vi "StartAlbumAcq.vi"(8 "error in (no error)":errorcluster, 11 "Config In":T1={"Hardware Configuration"={"Camera Configuration"={"Setting"={"Expouse"=0.0, "Frames"=0.0, "Interval"=0.0, "ROI"={"x"=0.0, "y"=0.0, "width"=0.0, "height"=0.0}, "Binning"={"Binning X"=0.0, "Binning Y"=0.0}}, "Resource"={"CameraRef"=refnum, "LibraryRef"=refnum, "ImagesArray"=[]}}, "Stages Configuration"={"Resource"={"NanoStage Ref"=0, "MicroStage Ref"=0, "TirfLock Ref"=0}, "SettingValues"={"NanoState"={"Time"=0.0, "X"=0.0, "Y"=0.0, "Z"=0.0}, "MicroState"={"Time 2"=0.0, "Z"=0.0, "IsEPISet?"=FALSE}, "TirfLock"={"Time"=0.0, "X"=0.0, "Y"=0.0, "Sum"=0.0, "Calbrate"=0.0, "LockedTarget"=0.0, "Kp"=0.0, "Ki"=0.0, "Avg"=0.0}}}, "Lasers Configuration"={"SettingValues"={"405 Power"=0.0, "488 Power"=0.0, "532 Power"=0.0, "561 Power"=0.0, "647 Power"=0.0, "785 Power"=0.0}, "Resource"={"Library Ref"=refnum, "Lasers Ref"={"405 Ref"=refnum, "488 Ref"=refnum, "532 Ref"=refnum, "561 Ref"=refnum, "647 Ref"=refnum, "785 Ref"=refnum}}}}, "Logging Configuration"={"Log File Base Folder"=path "", "FileSurfix"="", "TiffFileFullPath"=path "", "TimeStampFile Ref"=refnum, "NoteFileRef"=refnum, "QuickNoteInfo"=""}, "HardWare Status"={"CameraAndStages"={"Camera"=FALSE, "NanoStage"=FALSE, "MicroStage"=FALSE, "TIRFLock"=FALSE}, "Lasers"={"IsConnected"={"405"=FALSE, "488"=FALSE, "532"=FALSE, "561"=FALSE, "647"=FALSE, "785"=FALSE}, "IsOpened"={"405"=FALSE, "488"=FALSE, "532"=FALSE, "561"=FALSE, "647"=FALSE, "785"=FALSE}}}, "CallBack Ref"={"LiveAcq callback Ref"=refnum, "AlbumAcq callback Ref"=refnum, "SequenceAcq callback Ref"=refnum, "Camera Status callback Ref"=refnum}, "Acqusition Control"={"Images Saving"={"StreamToDisk?"=FALSE, "SingleStack?"=FALSE, "Alert when finish?"=FALSE}, "Debug"={"Global Debug"=FALSE, "Global Debug Value"=0.0}}, "Runtime Parameters"={"Scale Bar"=TRUE, "ScaleBarSize"=10.0, "XYIncreatement+"=40.0, "ZIncreatement++"=5.0, "Autostretch"=FALSE, "ZIncreatement+"=0.2, "MicroStage+"=100.0, "XYIncreatement++"=80.0}} {"Runtime Parameters"."XYIncreatement++" format="%#_13g"; "Runtime Parameters"."MicroStage+" format="%#_13g"; "Runtime Parameters"."ZIncreatement+" format="%#_13g"; "Runtime Parameters"."ZIncreatement++" format="%#_13g"; "Runtime Parameters"."XYIncreatement+" format="%#_13g"; "Runtime Parameters"."ScaleBarSize" format="%#_13g"; "Hardware Configuration"."Lasers Configuration"."SettingValues"."785 Power" format="%.1f"; "Hardware Configuration"."Lasers Configuration"."SettingValues"."647 Power" format="%.1f"; "Hardware Configuration"."Lasers Configuration"."SettingValues"."561 Power" format="%.1f"}) -> (0 "error out":errorcluster, 3 "Config Out":T1={"Hardware Configuration"={"Camera Configuration"={"Setting"={"Expouse"=0.0, "Frames"=0.0, "Interval"=0.0, "ROI"={"x"=0.0, "y"=0.0, "width"=0.0, "height"=0.0}, "Binning"={"Binning X"=0.0, "Binning Y"=0.0}}, "Resource"={"CameraRef"=refnum, "LibraryRef"=refnum, "ImagesArray"=[]}}, "Stages Configuration"={"Resource"={"NanoStage Ref"=0, "MicroStage Ref"=0, "TirfLock Ref"=0}, "SettingValues"={"NanoState"={"Time"=0.0, "X"=0.0, "Y"=0.0, "Z"=0.0}, "MicroState"={"Time 2"=0.0, "Z"=0.0, "IsEPISet?"=FALSE}, "TirfLock"={"Time"=0.0, "X"=0.0, "Y"=0.0, "Sum"=0.0, "Calbrate"=0.0, "LockedTarget"=0.0, "Kp"=0.0, "Ki"=0.0, "Avg"=0.0}}}, "Lasers Configuration"={"SettingValues"={"405 Power"=0.0, "488 Power"=0.0, "532 Power"=0.0, "561 Power"=0.0, "647 Power"=0.0, "785 Power"=0.0}, "Resource"={"Library Ref"=refnum, "Lasers Ref"={"405 Ref"=refnum, "488 Ref"=refnum, "532 Ref"=refnum, "561 Ref"=refnum, "647 Ref"=refnum, "785 Ref"=refnum}}}}, "Logging Configuration"={"Log File Base Folder"=path "", "FileSurfix"="", "TiffFileFullPath"=path "", "TimeStampFile Ref"=refnum, "NoteFileRef"=refnum, "QuickNoteInfo"=""}, "HardWare Status"={"CameraAndStages"={"Camera"=FALSE, "NanoStage"=FALSE, "MicroStage"=FALSE, "TIRFLock"=FALSE}, "Lasers"={"IsConnected"={"405"=FALSE, "488"=FALSE, "532"=FALSE, "561"=FALSE, "647"=FALSE, "785"=FALSE}, "IsOpened"={"405"=FALSE, "488"=FALSE, "532"=FALSE, "561"=FALSE, "647"=FALSE, "785"=FALSE}}}, "CallBack Ref"={"LiveAcq callback Ref"=refnum, "AlbumAcq callback Ref"=refnum, "SequenceAcq callback Ref"=refnum, "Camera Status callback Ref"=refnum}, "Acqusition Control"={"Images Saving"={"StreamToDisk?"=FALSE, "SingleStack?"=FALSE, "Alert when finish?"=FALSE}, "Debug"={"Global Debug"=FALSE, "Global Debug Value"=0.0}}, "Runtime Parameters"={"Scale Bar"=TRUE, "ScaleBarSize"=10.0, "XYIncreatement+"=40.0, "ZIncreatement++"=5.0, "Autostretch"=FALSE, "ZIncreatement+"=0.2, "MicroStage+"=100.0, "XYIncreatement++"=80.0}} {"Runtime Parameters"."XYIncreatement++" format="%#_13g"; "Runtime Parameters"."MicroStage+" format="%#_13g"; "Runtime Parameters"."ZIncreatement+" format="%#_13g"; "Runtime Parameters"."ZIncreatement++" format="%#_13g"; "Runtime Parameters"."XYIncreatement+" format="%#_13g"; "Runtime Parameters"."ScaleBarSize" format="%#_13g"; "Hardware Configuration"."Lasers Configuration"."SettingValues"."785 Power" format="%.1f"; "Hardware Configuration"."Lasers Configuration"."SettingValues"."647 Power" format="%.1f"; "Hardware Configuration"."Lasers Configuration"."SettingValues"."561 Power" format="%.1f"})   [LabVIEW 2020]
uses:
  Settings/System Running Settings.ctl
  Support/Hardware Configuration.ctl
  Support/Camera Configuration.ctl
  controls/ROI.ctl
  D:/Daguan/Development/RM21-MMicrosopeSource/HardwareAdapter/Camera/Dependencies/PVCamNET.dll
  Dependencies/PVCamNET.dll
  <vilib>/vision/Image Controls.llb/IMAQ Image.ctl
  D:/Daguan/Development/RM21-MMicrosopeSource/HardwareAdapter/Lasers/Dependencies/Oxxius_Boxx.dll
  Lasers/Dependencies/Oxxius_Boxx.dll
  Logging/Logging Configuration.ctl
  controls/DeviceStatusCtl.ctl
  controls/CallBack Refs.ctl
  Acquisition/Acquisition Control.ctl
  controls/Runtime Parameters.ctl
  Global.vi
  Logging/Logging.lvlib
  Settings/Settings.lvlib
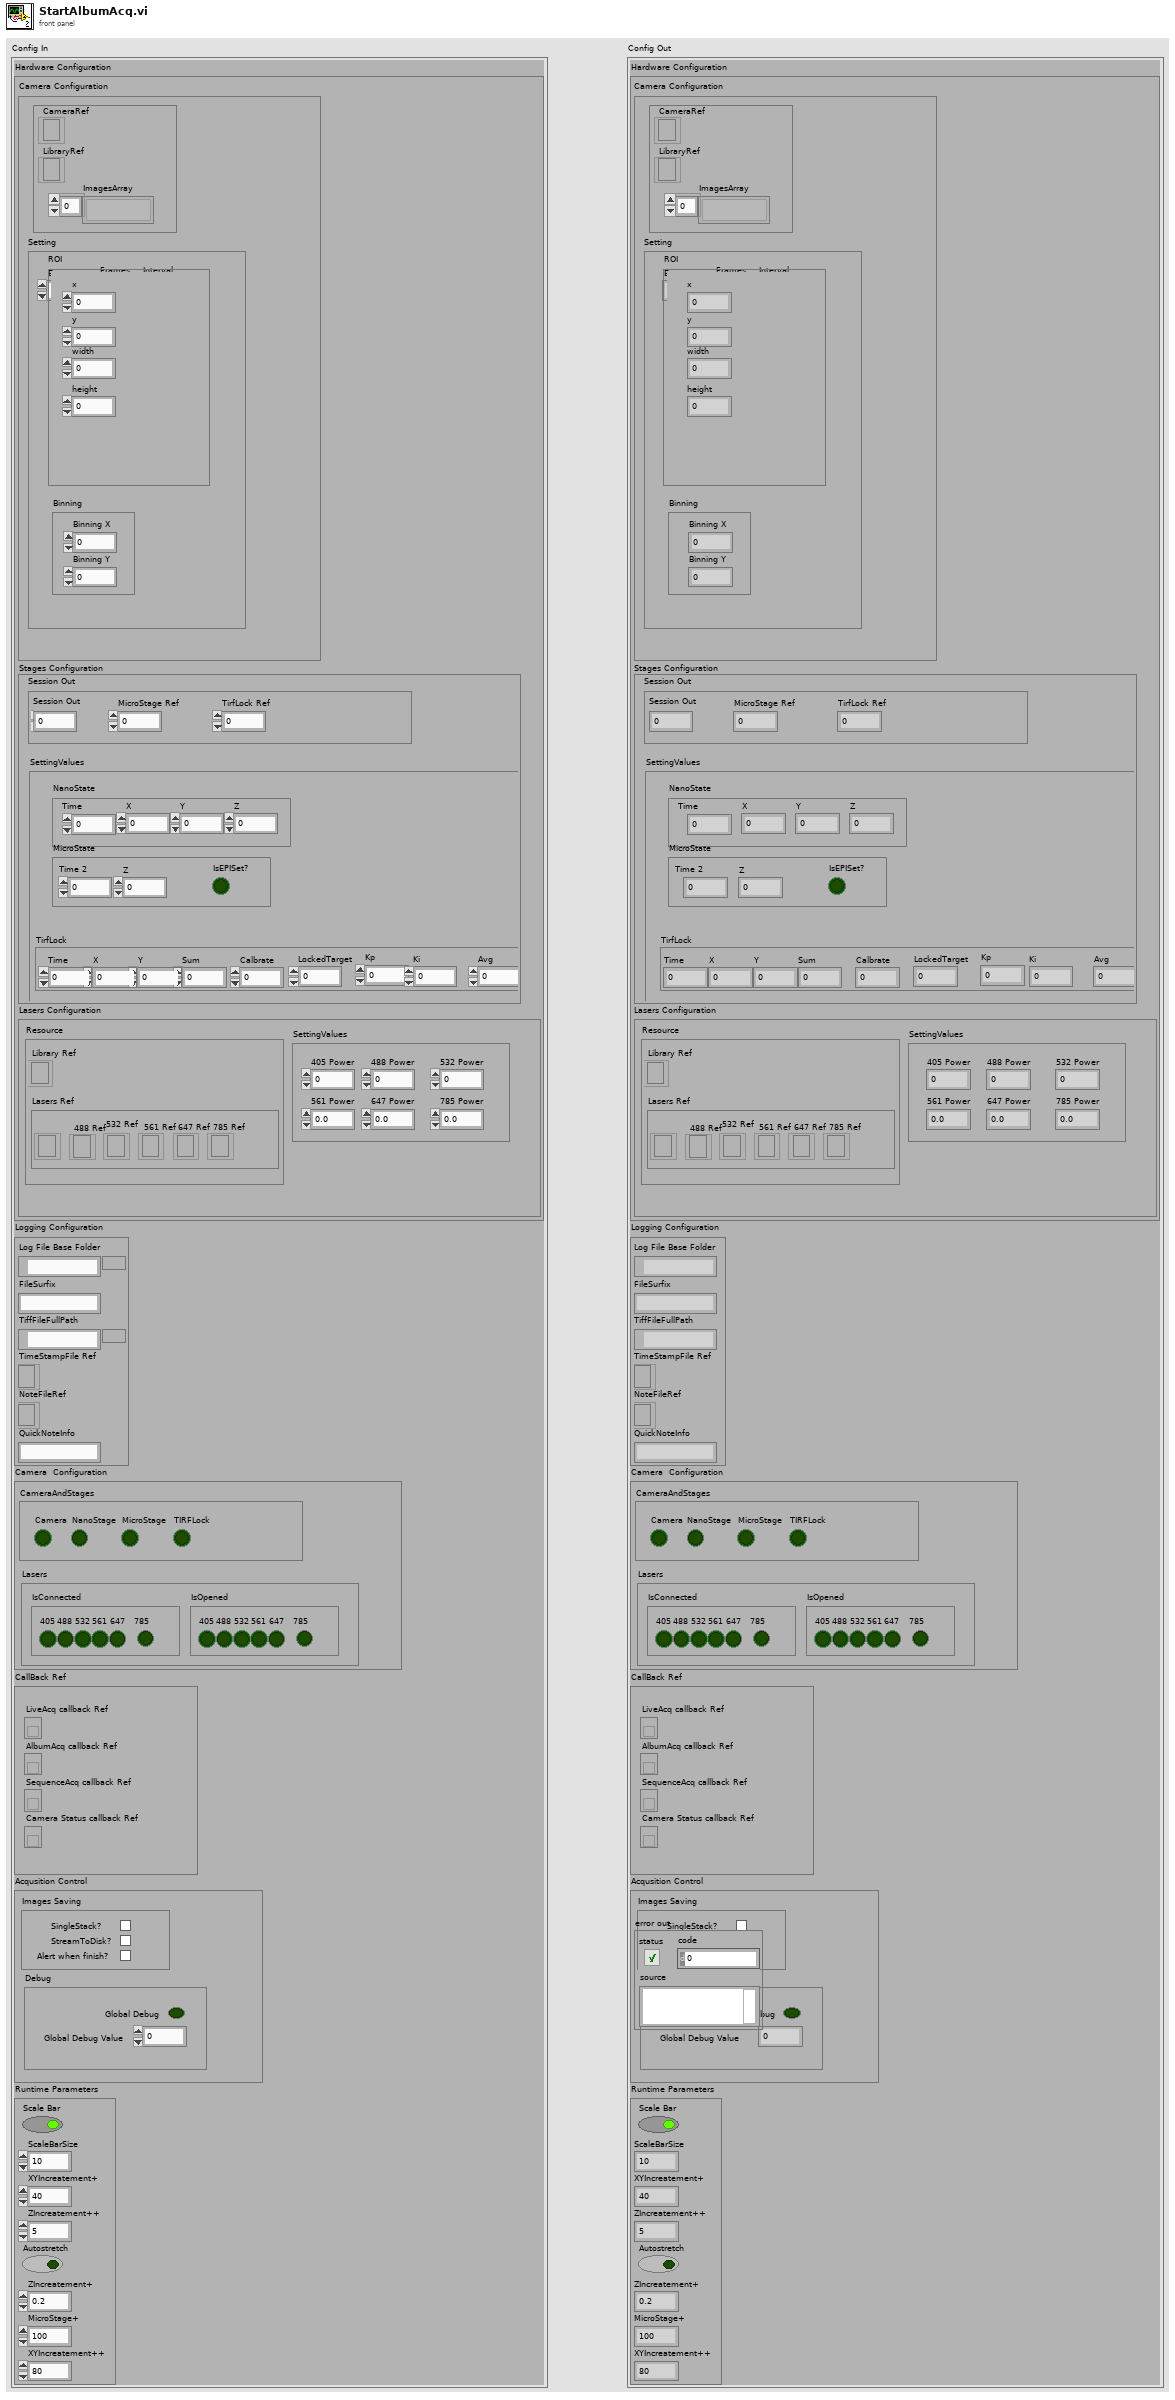
[diagram p1: front panel]
types:
  T1 = typedef "Settings.lvlib/System Running Settings.ctl" = cluster{"Hardware Configuration":T2, "Logging Configuration":T6, "HardWare Status":cluster{"CameraAndStages":T7, "Lasers":cluster{"IsConnected":cluster{"405":bool, "488":bool, "532":bool, "561":bool, "647":bool, "785":bool}, "IsOpened":cluster{"405":bool, "488":bool, "532":bool, "561":bool, "647":bool, "785":bool}}}, "CallBack Ref":T8, "Acqusition Control":T9, "Runtime Parameters":T10}
  T2 = typedef "Hardware Configuration.ctl" = cluster{"Camera Configuration":T3, "Stages Configuration":cluster{"Resource":cluster{"NanoStage Ref":i32, "MicroStage Ref":i32, "TirfLock Ref":i32}, "SettingValues":cluster{"NanoState":cluster{"Time":dbl, "X":dbl, "Y":dbl, "Z":dbl}, "MicroState":cluster{"Time 2":dbl, "Z":dbl, "IsEPISet?":bool}, "TirfLock":cluster{"Time":dbl, "X":dbl, "Y":dbl, "Sum":dbl, "Calbrate":dbl, "LockedTarget":dbl, "Kp":dbl, "Ki":dbl, "Avg":dbl}}}, "Lasers Configuration":cluster{"SettingValues":cluster{"405 Power":sgl, "488 Power":sgl, "532 Power":sgl, "561 Power":sgl, "647 Power":sgl, "785 Power":sgl}, "Resource":cluster{"Library Ref":refnum<k24>, "Lasers Ref":cluster{"405 Ref":refnum<k24>, "488 Ref":refnum<k24>, "532 Ref":refnum<k24>, "561 Ref":refnum<k24>, "647 Ref":refnum<k24>, "785 Ref":refnum<k24>}}}}
  T3 = typedef "Camera Configuration.ctl" = cluster{"Setting":cluster{"Expouse":dbl, "Frames":dbl, "Interval":dbl, "ROI":T4, "Binning":cluster{"Binning X":dbl, "Binning Y":dbl}}, "Resource":cluster{"CameraRef":refnum<k24>, "LibraryRef":refnum<k24>, "ImagesArray":T5[]}}
  T4 = typedef "ROI.ctl" = cluster{"x":dbl, "y":dbl, "width":dbl, "height":dbl}
  T5 = typedef "IMAQ Image.ctl" = refnum<image>
  T6 = typedef "Logging.lvlib/Logging Configuration.ctl" = cluster{"Log File Base Folder":path, "FileSurfix":string, "TiffFileFullPath":path, "TimeStampFile Ref":refnum<file>, "NoteFileRef":refnum<file>, "QuickNoteInfo":string}
  T7 = typedef "DeviceStatusCtl.ctl" = cluster{"Camera":bool, "NanoStage":bool, "MicroStage":bool, "TIRFLock":bool}
  T8 = typedef "CallBack Refs.ctl" = cluster{"LiveAcq callback Ref":refnum<k27>, "AlbumAcq callback Ref":refnum<k27>, "SequenceAcq callback Ref":refnum<k27>, "Camera Status callback Ref":refnum<k27>}
  T9 = typedef "Acquisition Control.ctl" = cluster{"Images Saving":cluster{"StreamToDisk?":bool, "SingleStack?":bool, "Alert when finish?":bool}, "Debug":cluster{"Global Debug":bool, "Global Debug Value":dbl}}
  T10 = typedef "Runtime Parameters.ctl" = cluster{"Scale Bar":bool, "ScaleBarSize":dbl, "XYIncreatement+":dbl, "ZIncreatement++":dbl, "Autostretch":bool, "ZIncreatement+":dbl, "MicroStage+":dbl, "XYIncreatement++":dbl}
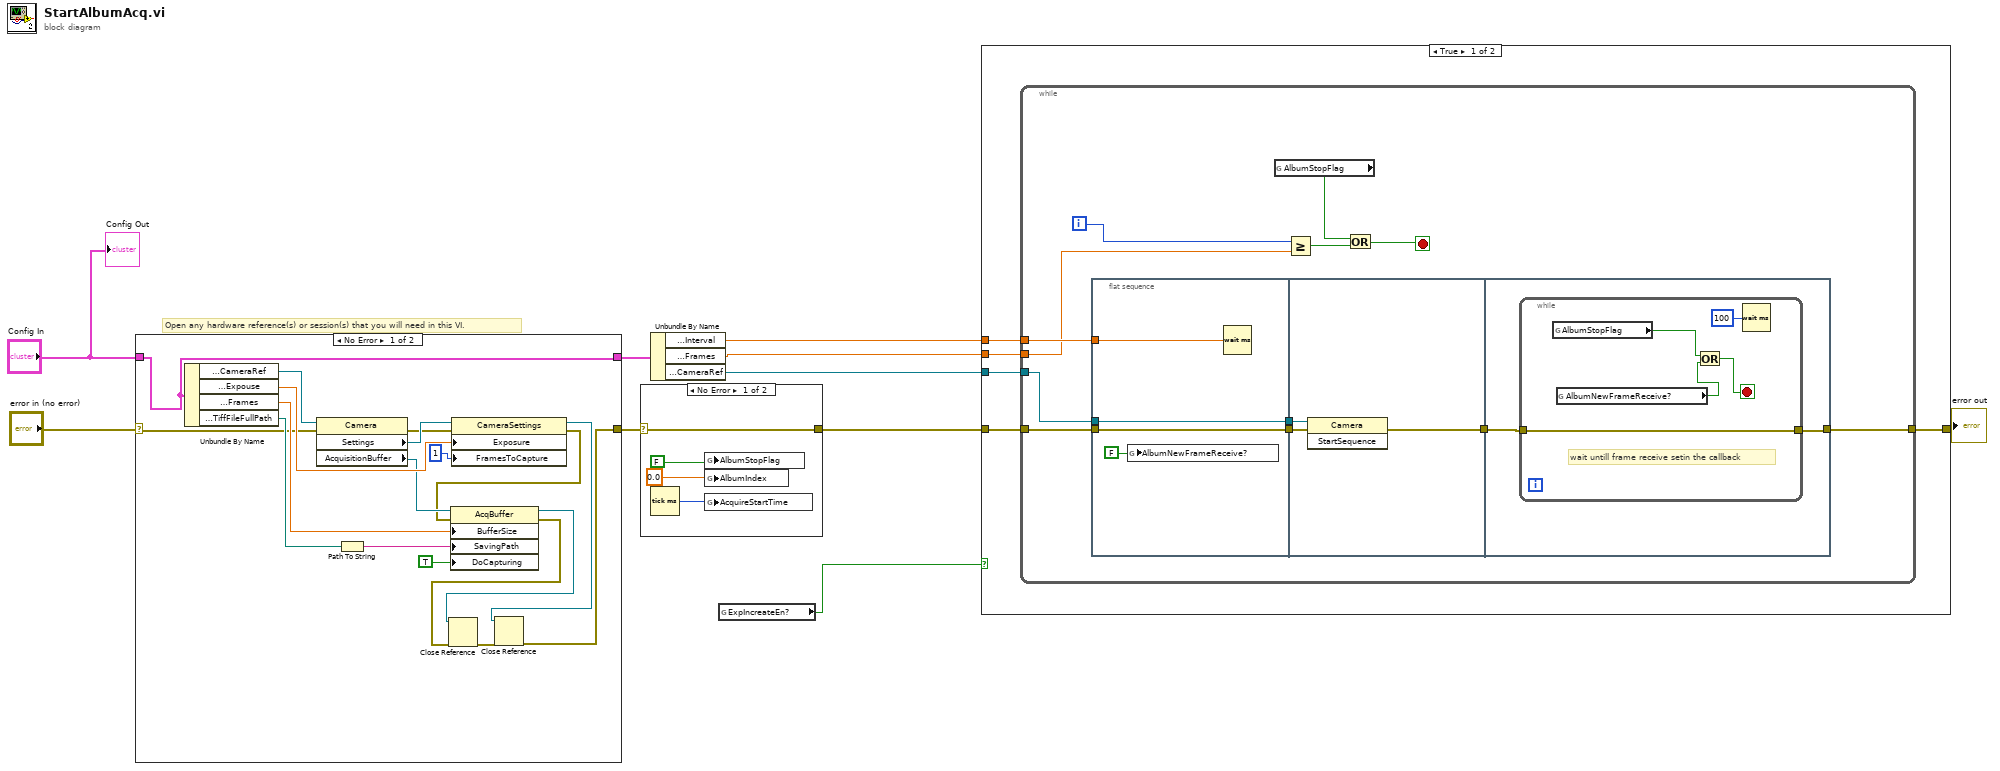
[diagram p0: block diagram]
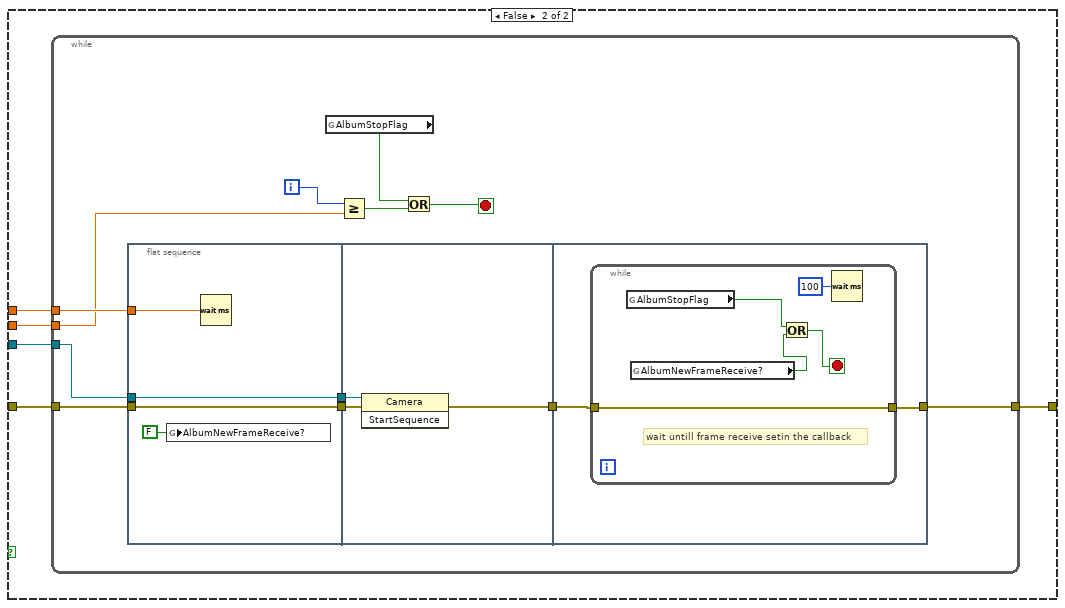
[diagram p2: hidden frame]
diagram:
  # "Open any hardware reference(s) or session(s) that you will need in this VI."
  n1 = case shown="No Error" "error in (no error)" {
    selector: "error in (no error)" -> [w24 w29]
    tunnel: [w13 w29] -> w5
    tunnel: "Config In" -> [w25 w30]
    tunnel: [w25 w30] -> w1
    frame No Error {
      n2 = Unbundle By Name(w25) -> ("Hardware Configuration.Camera Configuration.Resource.CameraRef"=w23:refnum<k24>, "Hardware Configuration.Camera Configuration.Setting.Expouse"=w28:dbl, "Hardware Configuration.Camera Configuration.Setting.Frames"=w27:dbl, "Logging Configuration.TiffFileFullPath"=w26:path)
      n3 = property class="Camera"(reference=w23, error in=w24) -> (error out=w21:errorcluster, "Settings"=w22:refnum<k24>, "AcquisitionBuffer"=w20:refnum<k24>)  [unwired: 1 out]
      n4 = Path To String(path=w26) -> (string=w18:string)
      n5 = property class="CameraSettings"(reference=w22, error in=w21, "Exposure"=w28, "FramesToCapture"=u16 1) -> (reference out=w12:refnum<k24>, error out=w19:errorcluster)
      n6 = property class="AcqBuffer"(reference=w20, error in=w19, "BufferSize"=w27, "SavingPath"=w18, "DoCapturing"=TRUE) -> (reference out=w11:refnum<k24>, error out=w15:errorcluster)
      n7 = Close Reference(reference=w11, error in (no error)=w15) -> (error out=w14:errorcluster)
      n8 = Close Reference(reference=w12, error in (no error)=w14) -> (error out=w13:errorcluster)
    }
    frame Error {
    }
  }
  n9 = case shown="No Error" w5 {
    selector: w5 -> [w31 w35]
    tunnel: [w31 w35] -> w4
    frame No Error {
      n10 = Tick Count (ms)() -> (millisecond timer value=w34:u32)
      n11 = global write "Global.vi" "AlbumStopFlag"(FALSE ("AlbumStopFlag")) -> ()
      n12 = global write "Global.vi" "AlbumIndex"(0.0 ("Albumndex")) -> ()
      n13 = global write "Global.vi" "AcquireStartTime"(w34) -> ()
    }
    frame Error {
    }
  }
  n14 = Unbundle By Name(w1) -> ("Hardware Configuration.Camera Configuration.Setting.Interval"=w9:dbl, "Hardware Configuration.Camera Configuration.Setting.Frames"=w7:dbl, "Hardware Configuration.Camera Configuration.Resource.CameraRef"=w6:refnum<k24>)
  n15 = global read "Global.vi" "ExpIncreateEn?"() -> (w3:bool)
  n16 = case shown="True" w3 {
    tunnel: w9 -> [w36 w67]
    tunnel: w7 -> [w38 w69]
    tunnel: w6 -> [w37 w68]
    tunnel: w4 -> [w40 w71]
    tunnel: [w39 w70] -> w2
    frame True {
      n17 = while {
        tunnel: w40 -> [w50]
        tunnel: [w43] -> w39
        tunnel: w38 -> [w41]
        tunnel: w37 -> [w48]
        tunnel: w36 -> [w42]
        i -> [w47]
        stop <- w49 stop-if-true
        n18 = flat-sequence {
          tunnel: w48 -> [w55]
          tunnel: w50 -> [w56]
          tunnel: [w56] -> w46
          tunnel: [w55] -> w45
          tunnel: w42 -> [w53]
          tunnel: w46 -> [w59]
          tunnel: w45 -> [w58]
          tunnel: [w57] -> w44
          tunnel: [w60] -> w43
          tunnel: w44 -> [w61]
          frame #0 {
            n19 = global write "Global.vi" "AlbumNewFrameReceive?"(FALSE ("AlbumNewFrameReceive?")) -> ()
            n20 = Wait (ms)(milliseconds to wait=w53) -> ()  [unwired: 1 out]
          }
          frame #1 {
            n21 = invoke class="Camera" method="StartSequence"(reference=w58, error in=w59) -> (error out=w57:errorcluster)  [unwired: 1 in, 2 out]
          }
          frame #2 {
            n22 = while {
              tunnel: [w65] -> w60
              tunnel: w61 -> [w65]
              stop <- w62 stop-if-true
              # "wait untill frame receive setin the callback"
              n23 = global read "Global.vi" "AlbumStopFlag"() -> (w64:bool)
              n24 = global read "Global.vi" "AlbumNewFrameReceive?"() -> (w63:bool)
              n25 = Or(x=w64, y=w63) -> (x .or. y?=w62:bool)
              n26 = Wait (ms)(milliseconds to wait=u32 100) -> ()  [unwired: 1 out]
            }
          }
        }
        n27 = global read "Global.vi" "AlbumStopFlag"() -> (w51:bool)
        n28 = Greater Or Equal?(x=w47, y=w41) -> (x >= y?=w52:bool)
        n29 = Or(x=w51, y=w52) -> (x .or. y?=w49:bool)
      }
    }
    frame False {
      n30 = while {
        tunnel: w71 -> [w81]
        tunnel: [w74] -> w70
        tunnel: w69 -> [w72]
        tunnel: w68 -> [w79]
        tunnel: w67 -> [w73]
        i -> [w78]
        stop <- w80 stop-if-true
        n31 = flat-sequence {
          tunnel: w79 -> [w86]
          tunnel: w81 -> [w87]
          tunnel: [w87] -> w77
          tunnel: [w86] -> w76
          tunnel: w73 -> [w84]
          tunnel: w77 -> [w90]
          tunnel: w76 -> [w89]
          tunnel: [w88] -> w75
          tunnel: [w91] -> w74
          tunnel: w75 -> [w92]
          frame #0 {
            n32 = global write "Global.vi" "AlbumNewFrameReceive?"(FALSE ("AlbumNewFrameReceive?")) -> ()
            n33 = Wait (ms)(milliseconds to wait=w84) -> ()  [unwired: 1 out]
          }
          frame #1 {
            n34 = invoke class="Camera" method="StartSequence"(reference=w89, error in=w90) -> (error out=w88:errorcluster)  [unwired: 1 in, 2 out]
          }
          frame #2 {
            n35 = while {
              tunnel: [w96] -> w91
              tunnel: w92 -> [w96]
              stop <- w93 stop-if-true
              # "wait untill frame receive setin the callback"
              n36 = global read "Global.vi" "AlbumStopFlag"() -> (w95:bool)
              n37 = global read "Global.vi" "AlbumNewFrameReceive?"() -> (w94:bool)
              n38 = Or(x=w95, y=w94) -> (x .or. y?=w93:bool)
              n39 = Wait (ms)(milliseconds to wait=u32 100) -> ()  [unwired: 1 out]
            }
          }
        }
        n40 = global read "Global.vi" "AlbumStopFlag"() -> (w82:bool)
        n41 = Greater Or Equal?(x=w78, y=w72) -> (x >= y?=w83:bool)
        n42 = Or(x=w82, y=w83) -> (x .or. y?=w80:bool)
      }
    }
  }
  "error out" <- w2
  "Config Out" <- "Config In"
